vi "SetParamsPeriod.vi"(8 "error in (no error)":errorcluster) -> (0 "error out":errorcluster)   [LabVIEW 2014]
uses:
  <vilib>/addons/database/_DB Variant To Data/Database Variant To Data.xnode
panel:
  in  "取消":bool
  in  "确定":bool
  in  "自动测试":dbl
  in  "单次测试":dbl
  in  "自定义测试":dbl
  in  "常温拷机":dbl
  in  "高温老练":dbl
  in  "温循":dbl
  # "设置采集周期(单位:ms)"
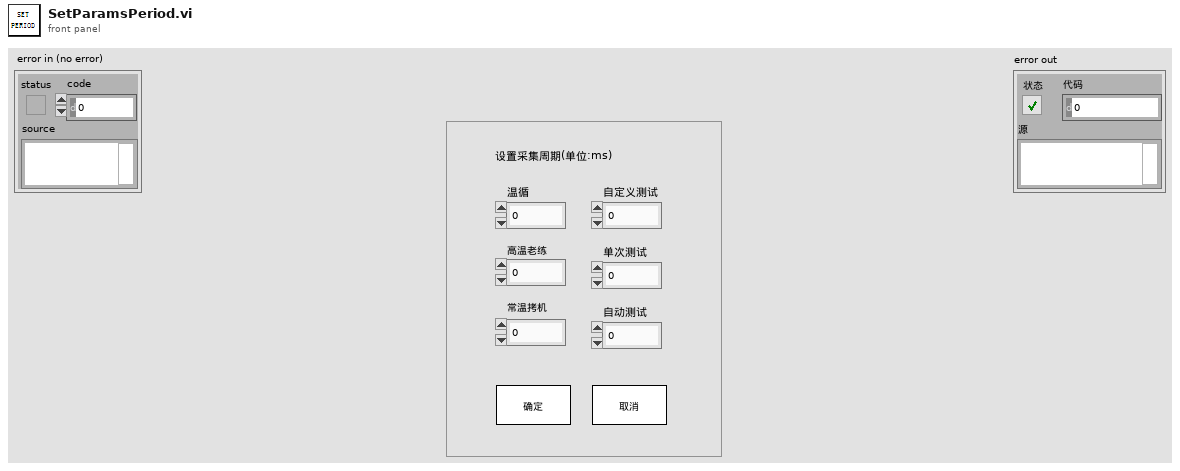
[diagram p1: front panel]
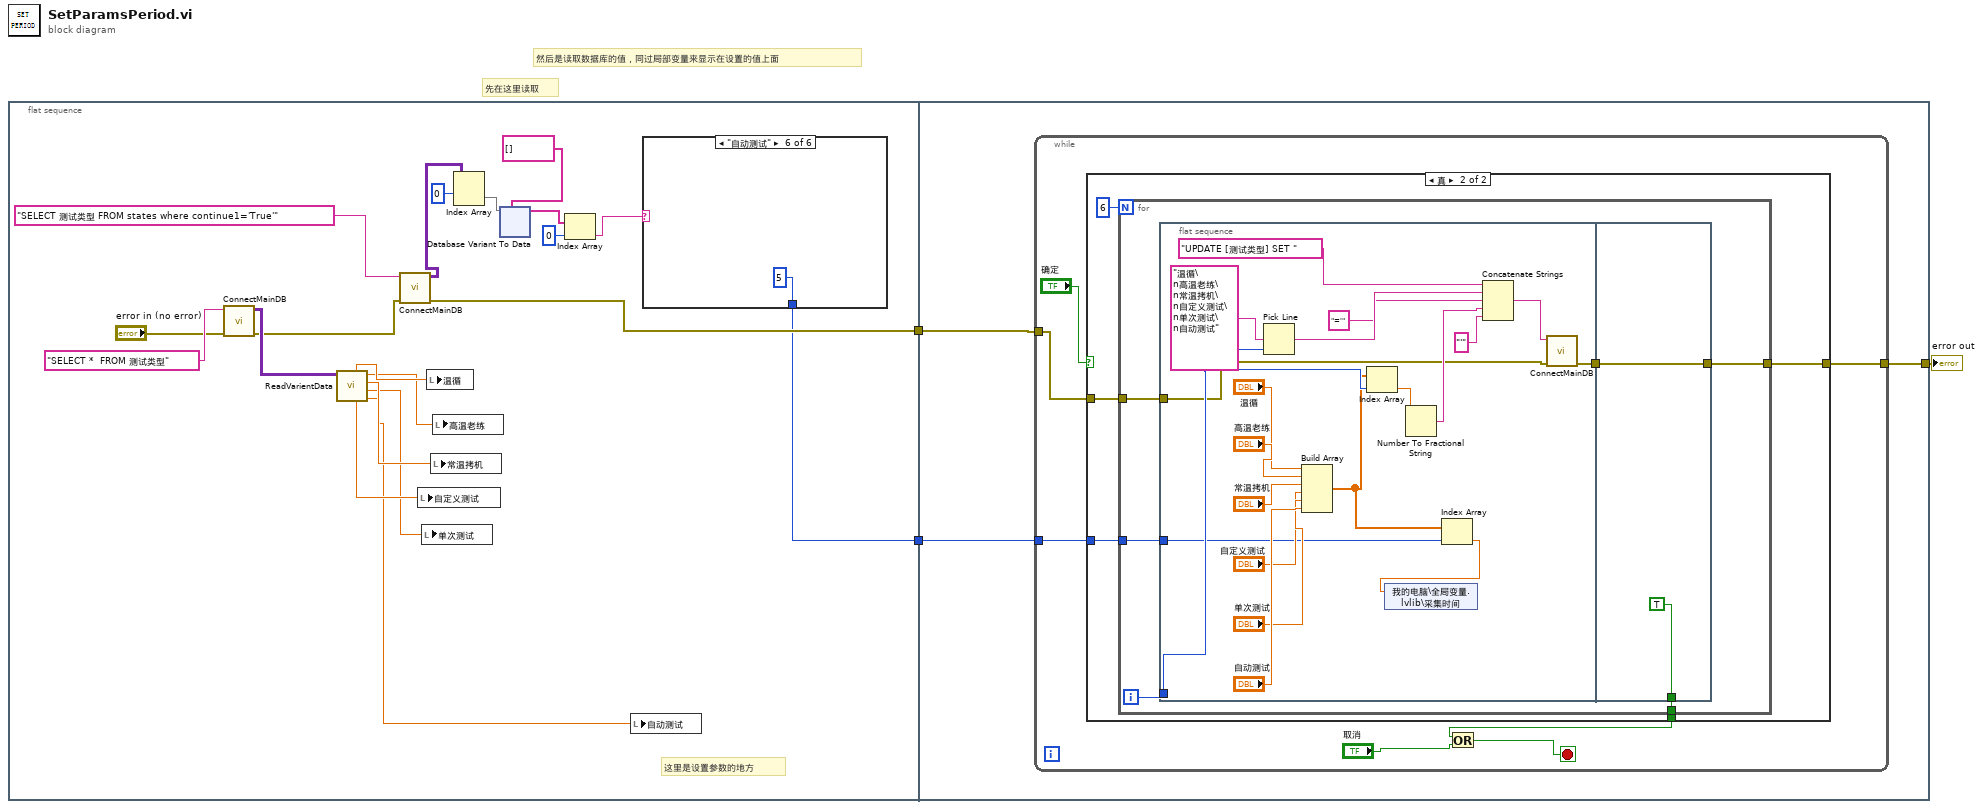
[diagram p0: block diagram]
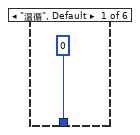
[diagram p2: hidden frame]
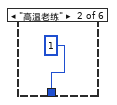
[diagram p3: hidden frame]
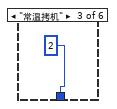
[diagram p4: hidden frame]
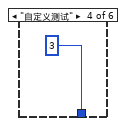
[diagram p5: hidden frame]
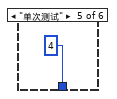
[diagram p6: hidden frame]
diagram:
  # "先在这里读取"
  # "然后是读取数据库的值，同过局部变量来显示在设置的值上面"
  n1 = flat-sequence {
    tunnel: [w13] -> w3
    tunnel: [w4] -> w1
    tunnel: w3 -> [w70]
    tunnel: [w69] -> w2
    tunnel: w1 -> [w68]
    frame #0 {
      # "这里是设置参数的地方"
      n2 = call "ConnectMainDB.vi"("error in (no error)"="error in (no error)", "SQL query"="SELECT *  FROM 测试类型") -> ("error out"=w14:errorcluster, "recordset data"=w15:variant[][])  [unwired: 8 in]
      n3 = call "ReadVarientData.vi"("数组"=w15) -> ("输出 6"=w18:dbl, "输出 5"=w19:dbl, "输出 3"=w21:dbl, "输出 2"=w22:dbl, "输出 4"=w20:dbl, "输出 1"=w23:dbl)  [unwired: 5 in]
      n4 = call "ConnectMainDB.vi"("error in (no error)"=w14, "SQL query"="SELECT 测试类型 FROM states where continue1='True'") -> ("error out"=w13:errorcluster, "recordset data"=w8:variant[][])  [unwired: 8 in]
      n5 = local write "自定义测试"(w20) -> ()
      n6 = local write "单次测试"(w19) -> ()
      n7 = local write "温循"(w23) -> ()
      n8 = local write "常温拷机"(w21) -> ()
      n9 = local write "高温老练"(w22) -> ()
      n10 = Index Array(array=w8, index (row)=0 ("索引 (行)")) -> (element=w10:variant[])  [unwired: 1 in]
      n11 = xnode "Database Variant To Data"("database variant"=w10, "type"=string[] []) -> ("data"=w6:string[])  [unwired: 1 in, 1 out]
      n12 = Index Array(array=w6, index=0 ("索引")) -> (element=w5:string)
      n13 = local write "自动测试"(w18) -> ()
      n14 = case shown="\"自动测试\"" w5 {
        tunnel: [0 1 2 3 4 5] -> w4
        frame "温循", Default {
        }
        frame "高温老练" {
        }
        frame "常温拷机" {
        }
        frame "自定义测试" {
        }
        frame "单次测试" {
        }
        frame "自动测试" {
        }
      }
    }
    frame #1 {
      n15 = while {
        tunnel: w70 -> [w74]
        tunnel: [w73] -> w69
        tunnel: w68 -> [w71]
        stop <- w76 stop-if-true
        n16 = case shown="真" "确定" {
          tunnel: w74 -> [_ w81]
          tunnel: [_ w80] -> w73
          tunnel: [_ w79] -> w72
          tunnel: w71 -> [_ w78]
          frame False {
          }
          frame True {
            n17 = for {
              N: 6 -> [_]
              tunnel: w81 -> [w87]
              tunnel: [w86] -> w80
              tunnel: [w84] -> w79
              tunnel: w78 -> [w83]
              i -> [w88]
              n18 = flat-sequence {
                tunnel: w88 -> [w99]
                tunnel: w87 -> [w93]
                tunnel: [w92] -> w85
                tunnel: w83 -> [w90]
                tunnel: [w110] -> w86
                tunnel: w85 -> [w110]
                tunnel: [TRUE] -> w84
                frame #0 {
                  n19 = Pick Line(multi-line string="温循\n高温老练\n常温拷机\n自定义测试\n单次测试\n自动测试" ("多行字符串"), line index=w99) -> (output string=w106:string)  [unwired: 1 in]
                  n20 = Build Array("温循", "高温老练", "常温拷机", "自定义测试", "单次测试", "自动测试") -> (w91:dbl[])
                  n21 = Index Array(array=w91, index=w99) -> (element=w97:dbl)
                  n22 = Number To Fractional String(number=w97) -> (F-format string=w96:string)  [unwired: 3 in]
                  n23 = Index Array(array=w91, index=w90) -> (element=w89:dbl)
                  n24 = shared-variable "我的电脑\\全局变量.lvlib\\采集时间"(w89) -> ()  [unwired: 1 in, 1 out]
                  n25 = Concatenate Strings("UPDATE [测试类型] SET ", w106, "='", w96, "'") -> (w94:string)
                  n26 = call "ConnectMainDB.vi"("error in (no error)"=w93, "SQL query"=w94) -> ("error out"=w92:errorcluster)  [unwired: 8 in, 1 out]
                }
                frame #1 {
                }
              }
            }
          }
        }
        n27 = Or(x=w72, y="取消") -> (x .or. y?=w76:bool)
      }
    }
  }
  "error out" <- w2
